vi "Simple Reader.vi"(8 "error in (no error)":errorcluster, 11 "Magnet in":refnum<class "Magnet.lvclass">) -> (0 "error out":errorcluster, 2 "Signals":dbl[](array[numeric]), 3 "Magnet out":refnum<class "Magnet.lvclass">)   [LabVIEW 2018, in "Magnet.lvclass"]
uses:
  Magnet.lvclass
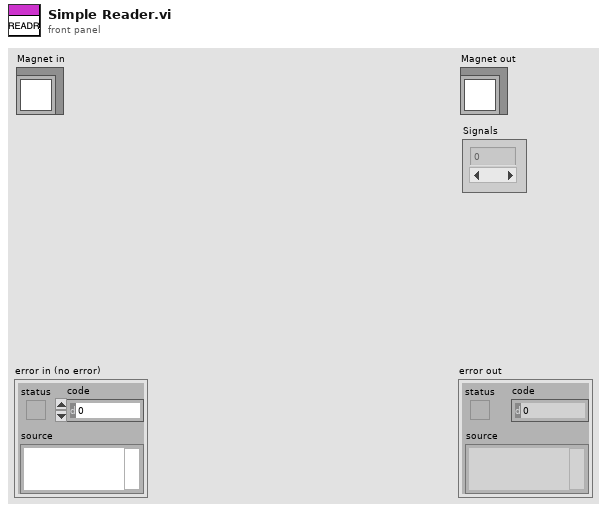
[diagram p1: front panel]
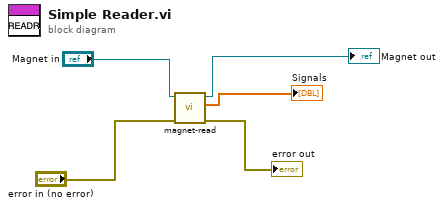
[diagram p0: block diagram]
diagram:
  n1 = call "magnet-read.vi"("error in (no error)"="error in (no error)", "magnet IN"="Magnet in") -> ("error out"=→"error out":errorcluster, "Result"=→"Signals":dbl[], "magnet OUT"=→"Magnet out":refnum<class "Magnet.lvclass">)  [unwired: 7 in]
